vi "fgv_inrange-lidar-data_buf.vi"(7 "cmd":enum16{"read", "write"}(ring), 10 "in range data new":T1(array[cluster]), 11 "in range data":cluster{sgl[], sgl[]}[](array[cluster])) -> (2 "in range data new out":T1(array[cluster]), 3 "in range data out":cluster{sgl[], sgl[]}[](array[cluster]))   [LabVIEW 2019]
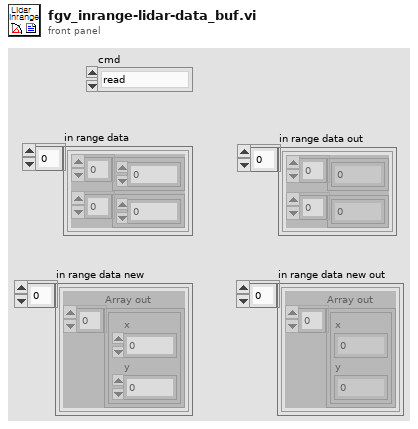
[diagram p1: front panel]
types:
  T1 = cluster{"Array out":cluster{"x":dbl, "y":dbl}[]}[]
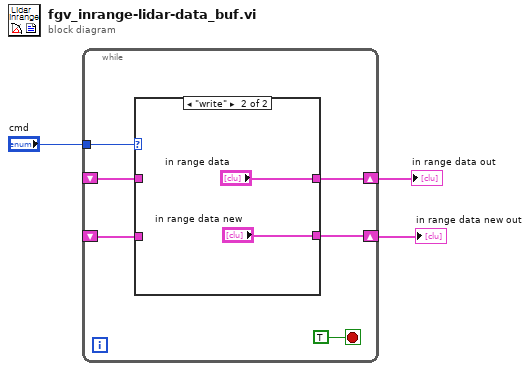
[diagram p0: block diagram]
diagram:
  n1 = while {
    tunnel: "cmd" -> [w8]
    shift-right: [w7] -> w2
    shift-left: _ -> [w6]
    shift-right: [w5] -> w1
    shift-left: _ -> [w4]
    stop <- TRUE stop-if-true
    n2 = case shown="\"write\"" w8 {
      tunnel: [w11 "in range data"] -> w7
      tunnel: w6 -> [w11 _]
      tunnel: [w10 "in range data new"] -> w5
      tunnel: w4 -> [w10 _]
      frame "read", Default {
      }
      frame "write" {
      }
    }
  }
  "in range data out" <- w2
  "in range data new out" <- w1
